vi "Periodic Tasks.vi"(8 "error in":errorcluster) -> ()   [LabVIEW 2012]
doc: "This VI runs in parallel to other tasks. It can contain as many user-defined periodic loops as you need. These can carry out PID or other sorts of timed response."
uses:
  <vilib>/Rock Robotics/SystemInterfaces/Utilities/FPGA_UtilitiesLED Source.ctl
  <vilib>/Rock Robotics/SystemInterfaces/Utilities/FPGA_UtilitiesLED State.ctl
  Robot Global Data.vi
  <vilib>/Rock Robotics/WPI/Compressor/WPI_CompressorGetSetRefNum.vi
  <vilib>/Rock Robotics/WPI/Joystick/WPI_JoystickGetSetRefNum.vi
  <vilib>/Rock Robotics/WPI/RobotDrive/WPI_RobotDriveGetSetRefNum.vi
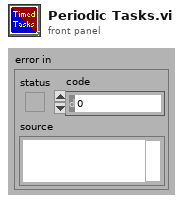
[diagram p1: front panel]
types:
  T1 = typedef "WPI_JoystickDevRef.ctl" = cluster{"Device":T2}
  T2 = typedef "WPI_JoystickDeviceEnum.ctl" = enum16{"USB 1", "USB 2", "USB 3", "USB 4", "Kinect 1", "Kinect 2"}
  T3 = typedef "WPI_RobotDriveDevRef.ctl" = cluster{"DevStatus":errorcluster, "Motors[]":T4[], "Square Inputs":bool, "Max Output":dbl, "Isochronous":bool}
  T4 = typedef "WPI_MotorControlDeviceRef.ctl" = cluster{"DeviceStatus":errorcluster, "Type":enum16{"PWM", "CAN"}, "PWM":cluster{"Digital Module":T5, "PWM Channel":T6, "DeadBand":T7}, "CAN":cluster{"Device Number":u8, "Control Mode":T8, "Semaphore":T9, "Max Vout":dbl}, "Invert":bool, "TransformRef":T10, "InvTransformRef":T10}
  T5 = typedef "FPGA_TypedefDigitalModule.ctl" = enum16{"Digital Module 1", "Digital Module 2"}
  T6 = typedef "FPGA_DIOPWMChannel.ctl" = enum8{"PWM 1", "PWM 2", "PWM 3", "PWM 4", "PWM 5", "PWM 6", "PWM 7", "PWM 8", "PWM 9", "PWM 10", "Invalid"}
  T7 = typedef "WPI_PWMDeadband.ctl" = cluster{"Name":string, "maxPositivePwm":i32, "minPositivePwm":i32, "centerPwm":i32, "maxNegativePwm":i32, "minNegativePwm":i32, "angularRange":u16}
  T8 = typedef "WPI_CANJaguar_ControlMode.ctl" = enum8{"Percent VBus", "Current", "Speed", "Position", "Voltage"}
  T9 = typedef "Semaphore RefNum" = refnum<k1>
  T10 = typedef "WPI_PWMTransform_ConPane.ctl" = refnum<vi>
  T11 = typedef "FPGA_WatchdogDevRef.ctl" = cluster{"DevStatus":errorcluster}
  T12 = cluster{"JoystickDevRef":T1, "RobotDriveDevRef":T3}
  T13 = typedef "FPGA_UtilitiesLED State.ctl" = enum16{"Off", "On", "Toggle"}
  T14 = typedef "FPGA_UtilitiesLED Source.ctl" = enum16{"User LED", "FPGA LED"}
  T15 = typedef "WPI_CompressorDevRef.ctl" = cluster{"DevStatus":errorcluster, "DigitalInputDevRef":T16, "RelayDevRef":T18}
  T16 = typedef "WPI_DigitalInputDevRef.ctl" = cluster{"DevStatus":errorcluster, "DIO Channel":T17, "Digital Module":T5}
  T17 = typedef "FPGA_DIOChannel.ctl" = enum8{"DIO 1", "DIO 2", "DIO 3", "DIO 4", "DIO 5", "DIO 6", "DIO 7", "DIO 8", "DIO 9", "DIO 10", "DIO 11", "DIO 12", "DIO 13", "DIO 14", "Invalid"}
  T18 = typedef "WPI_RelayDevRef.ctl" = cluster{"DevStatus":errorcluster, "Relay Channel":T19, "Digital Module":T5, "Relay Direction":T20}
  T19 = typedef "FPGA_DIORelayChannel.ctl" = enum8{"Relay 1", "Relay 2", "Relay 3", "Relay 4", "Relay 5", "Relay 6", "Relay 7", "Relay 8", "Invalid"}
  T20 = typedef "WPI_RelayDirection.ctl" = enum16{"Both directions", "Forward only", "Reverse only"}
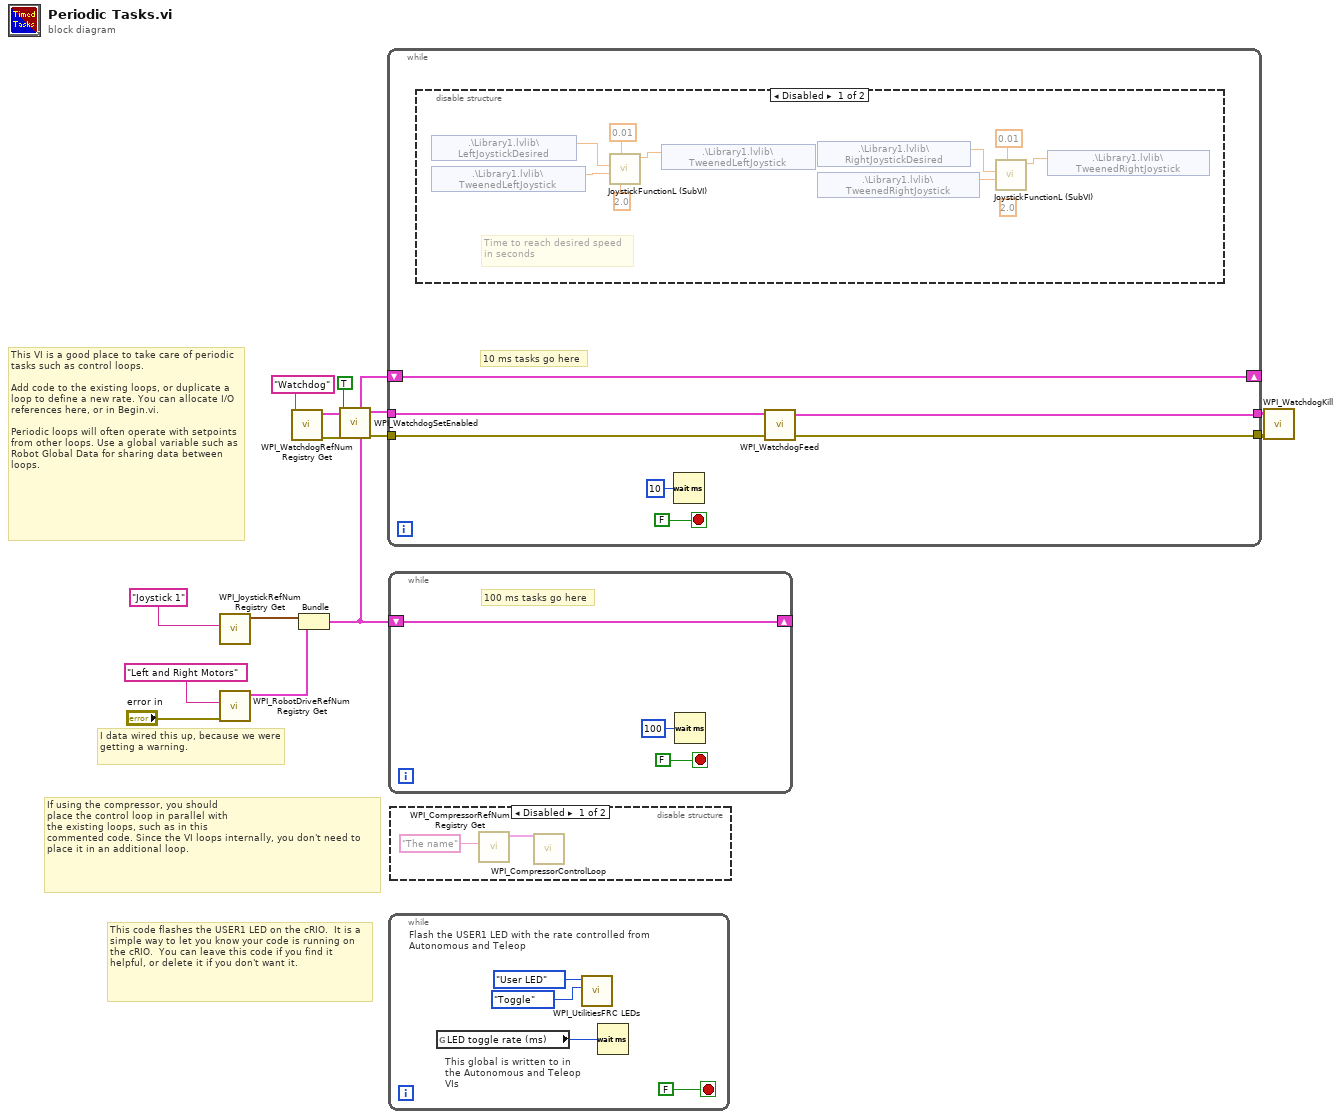
[diagram p0: block diagram]
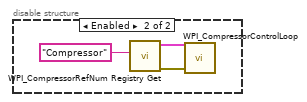
[diagram p2: hidden frame]
diagram:
  # "I data wired this up, because we were getting a warning."
  # "This VI is a good place to take care of periodic tasks such as control loops.\n\nAdd code to the existing loops, or duplicate a loop to define a new rate. You can allocate I/O references here, or in Begin.vi.\n\nPeriodic loops will often operate with setpoints from other loops. Use a global variable such as Robot Global Data for sharing data between loops."
  # "If using the compressor, you should\nplace the control loop in parallel with\nthe existing loops, such as in this\ncommented code. Since the VI loops internally, you don't need to place it in an additional loop."
  # "This code flashes the USER1 LED on the cRIO.  It is a simple way to let you know your code is running on the cRIO.  You can leave this code if you find it helpful, or delete it if you don't want it."
  n1 = call <vilib>:"WPI_JoystickRefNum Registry Get.vi"("refnum name"="Joystick 1") -> ("JoystickDevRef"=w12:T1)  [unwired: 1 in, 9 out]
  n2 = call <vilib>:"WPI_RobotDriveRefNum Registry Get.vi"("error in (no error)"="error in", "refnum name"="Left and Right Motors") -> ("RobotDriveDevRef"=w11:T3)  [unwired: 9 out]
  n3 = call <vilib>:"WPI_WatchdogRefNum Registry Get.vi"("refnum name"="Watchdog") -> ("error out"=w5:errorcluster, "WatchdogDevRef"=w8:T11)  [unwired: 9 in]
  n4 = Bundle("JoystickDevRef"=w12, "RobotDriveDevRef"=w11) -> (w10:T12)  [unwired: 1 out]
  n5 = call <vilib>:"WPI_WatchdogSetEnabled.vi"("error in (no error)"=w5, "Enabled"=TRUE, "WatchdogDevRef"=w8) -> ("error out"=w4:errorcluster, "WatchdogDevRef"=w7:T11)  [unwired: 7 in]
  n6 = while {
    shift-right: [w19] -> _
    shift-left: w10 -> [w19]
    tunnel: w7 -> [w18]
    tunnel: w4 -> [w17]
    tunnel: [w16] -> w2
    tunnel: [w15] -> w3
    stop <- FALSE stop-if-true
    # "10 ms tasks go here"
    n7 = disable-structure shown="Disabled" {
      frame Disabled {
        (unwired) 2.0 ("y")
        # "Time to reach desired speed\nin seconds"
        n8 = shared-variable ".\\Library1.lvlib\\LeftJoystickDesired"() -> (w29:dbl)  [unwired: 1 in, 1 out]
        n9 = shared-variable ".\\Library1.lvlib\\TweenedLeftJoystick"() -> (w30:dbl)  [unwired: 1 in, 1 out]
        n10 = call "JoystickFunctionL (SubVI).vi"("TimeToReachSpeed"=2.0 ("y"), "DeltaT"=0.01 ("y"), "TweenedSpeed"=w30, "DesiredSpeed"=w29) -> ("TweenedJoystick"=w28:dbl)  [unwired: 7 in]
        n11 = shared-variable ".\\Library1.lvlib\\TweenedLeftJoystick"(w28) -> ()  [unwired: 1 in, 1 out]
        n12 = shared-variable ".\\Library1.lvlib\\RightJoystickDesired"() -> (w23:dbl)  [unwired: 1 in, 1 out]
        n13 = shared-variable ".\\Library1.lvlib\\TweenedRightJoystick"() -> (w22:dbl)  [unwired: 1 in, 1 out]
        n14 = call "JoystickFunctionL (SubVI).vi"("DeltaT"=0.01 ("y"), "TweenedSpeed"=w22, "DesiredSpeed"=w23) -> ("TweenedJoystick"=w24:dbl)  [unwired: 8 in]
        n15 = shared-variable ".\\Library1.lvlib\\TweenedRightJoystick"(w24) -> ()  [unwired: 1 in, 1 out]
      }
      frame Enabled {
      }
    }
    n16 = Wait (ms)(milliseconds to wait=u32 10) -> ()  [unwired: 1 out]
    n17 = call <vilib>:"WPI_WatchdogFeed.vi"("error in (no error)"=w17, "WatchdogDevRef"=w18) -> ("error out"=w16:errorcluster, "WatchdogDevRef"=w15:T11)  [unwired: 8 in]
  }
  n18 = while {
    shift-right: [w31] -> _
    shift-left: w10 -> [w31]
    stop <- FALSE stop-if-true
    # "100 ms tasks go here"
    n19 = Wait (ms)(milliseconds to wait=u32 100) -> ()  [unwired: 1 out]
  }
  n20 = while {
    stop <- FALSE stop-if-true
    # "This global is written to in the Autonomous and Teleop VIs"
    # "Flash the USER1 LED with the rate controlled from Autonomous and Teleop"
    n21 = global read "Robot Global Data.vi" "LED toggle rate (ms)"() -> (w34:u32)
    n22 = call <vilib>:"WPI_UtilitiesFRC LEDs.vi"("State"=FPGA_UtilitiesLED_State."Toggle", "LED Type"=FPGA_UtilitiesLED_Source."User LED") -> ()  [unwired: 1 in, 9 out]
    n23 = Wait (ms)(milliseconds to wait=w34) -> ()  [unwired: 1 out]
  }
  n24 = disable-structure shown="Disabled" {
    frame Disabled {
      n25 = call <vilib>:"WPI_CompressorRefNum Registry Get.vi"("refnum name"="The name") -> ("CompressorDevRef"=w39:T15)  [unwired: 9 in, 1 out]
      n26 = call <vilib>:"WPI_CompressorControlLoop.vi"("CompressorDevRef"=w39) -> ()  [unwired: 11 in]
    }
    frame Enabled {
      n27 = call <vilib>:"WPI_CompressorRefNum Registry Get.vi"("refnum name"="Compressor") -> ("error out"=w40:errorcluster, "CompressorDevRef"=w42:T15)  [unwired: 9 in]
      n28 = call <vilib>:"WPI_CompressorControlLoop.vi"("error in (no error)"=w40, "CompressorDevRef"=w42) -> ()  [unwired: 10 in]
    }
  }
  n29 = call <vilib>:"WPI_WatchdogKill.vi"("error in (no error)"=w2, "WatchdogDevRef"=w3) -> ()  [unwired: 8 in, 2 out]
